vi "ClassSelectMess.vi"(7 "NewFunction":string, 8 "ErrorIn(No Error)":errorcluster caption="entrée d'erreur (pas d'erreur)", 9 "Text":string[][](array[string]), 10 "Functions":string[][](array[string]), 11 "Classes":string[][](array[string])) -> (0 "sortie d'erreur":errorcluster, 1 "CancelOut":bool, 2 "New":bool, 3 "InstrNameOut":string, 4 "Classindex":i32)   [LabVIEW 2019]
panel:
  out "Init Prog":bool
  in  "Cancel":bool
  in  "New":bool
  in  "Add":bool
  in  "LoadedDev":string(tree)
  # "Select an Instrument to add the function to or choose \"New\" to create the function into a new instrument"
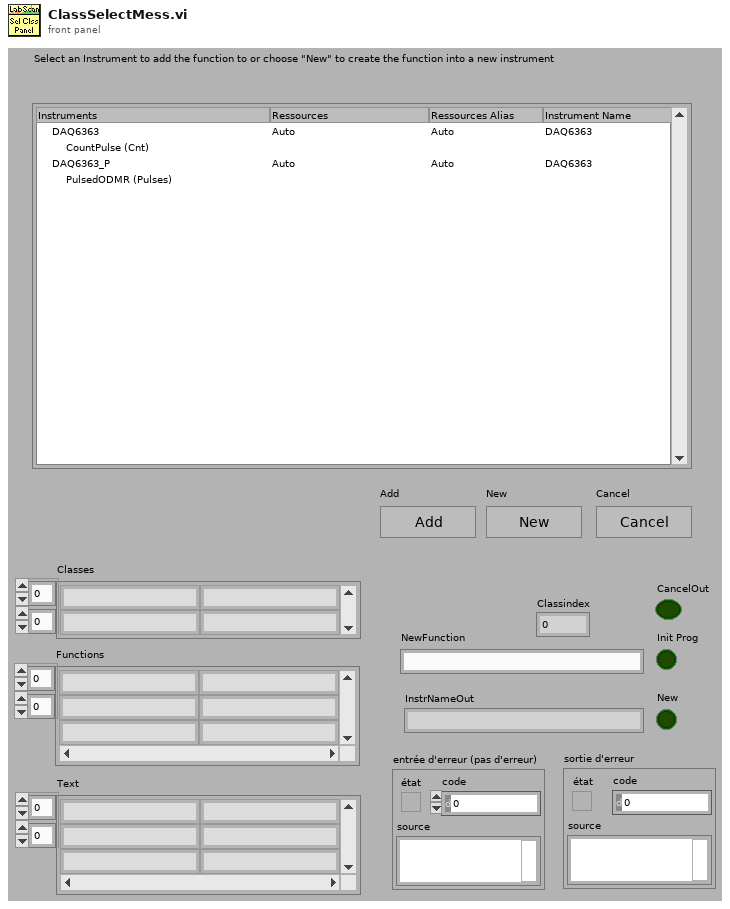
[diagram p1: front panel]
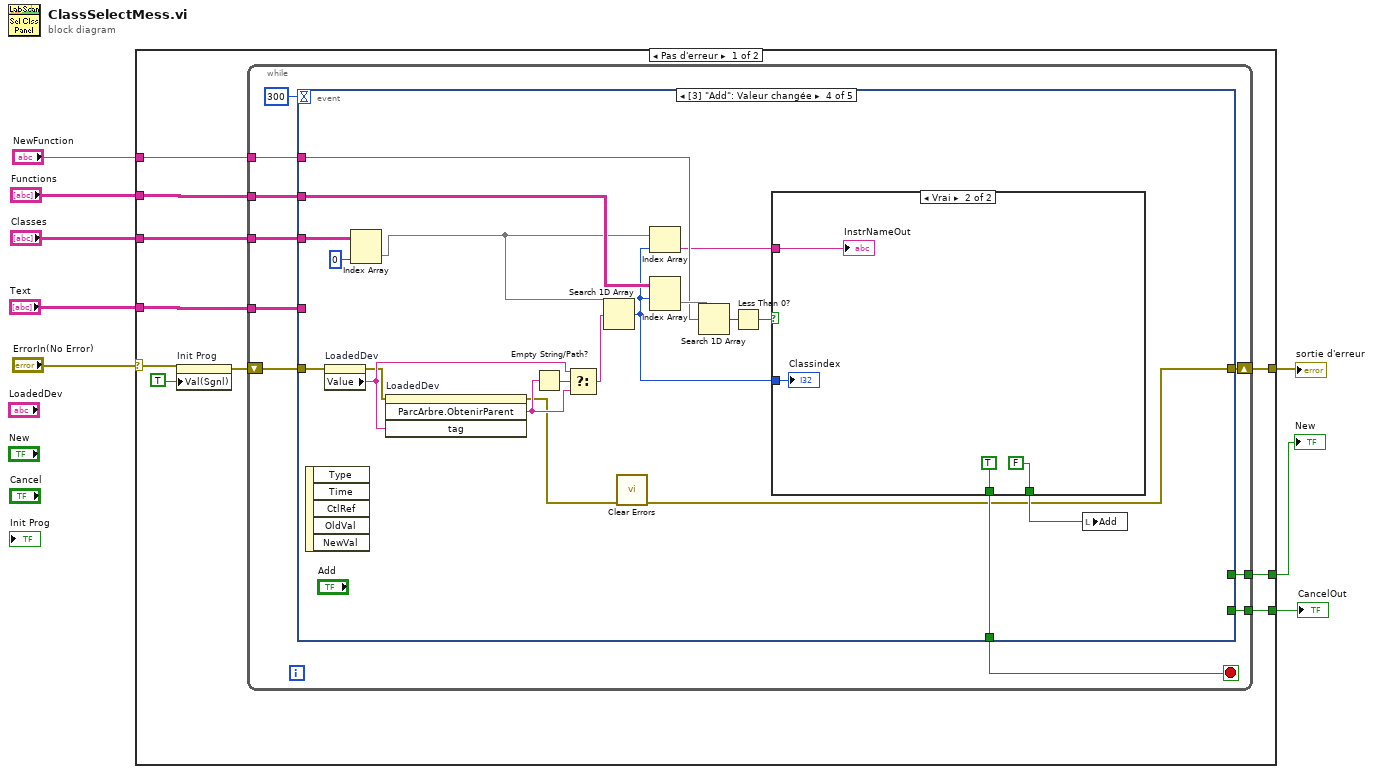
[diagram p0: block diagram]
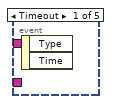
[diagram p2: hidden frame]
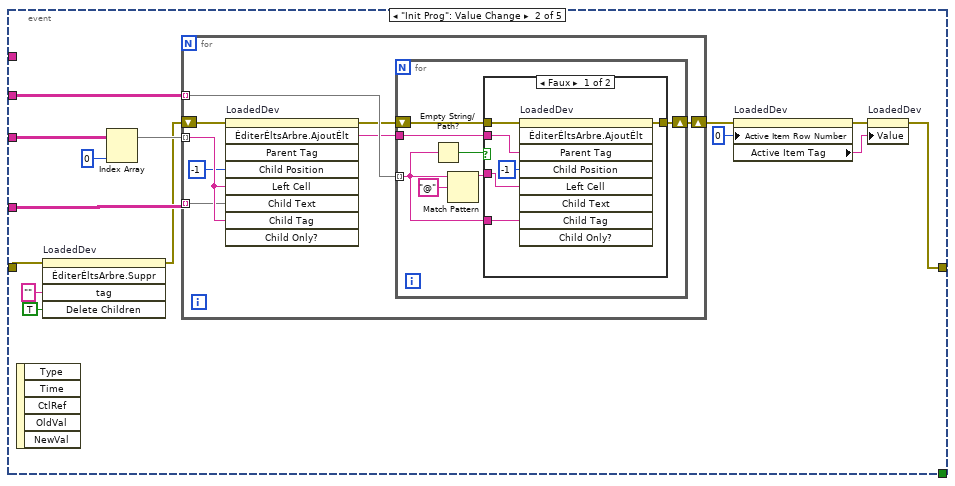
[diagram p3: hidden frame]
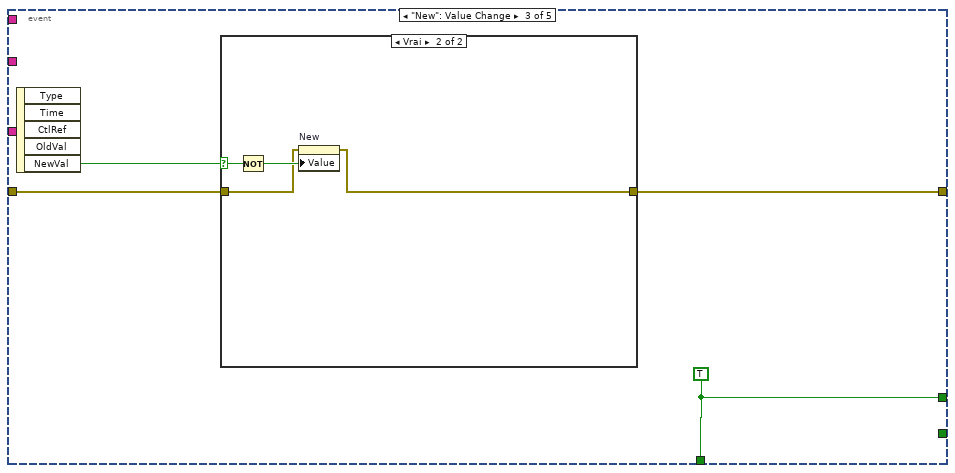
[diagram p5: hidden frame]
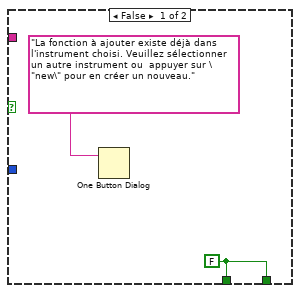
[diagram p7: hidden frame]
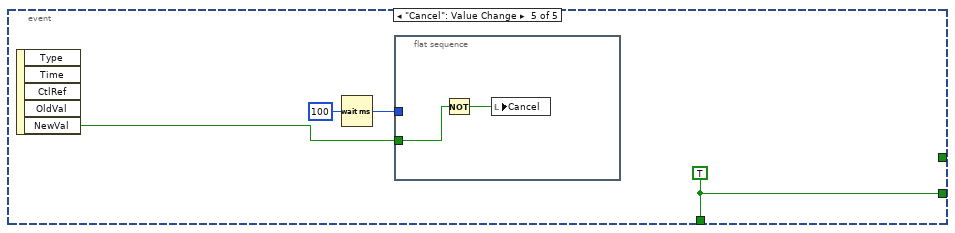
[diagram p8: hidden frame]
diagram:
  n1 = case shown="Pas d'erreur" "ErrorIn(No Error)" {
    selector: "ErrorIn(No Error)" -> [w14 w106]
    tunnel: "Classes" -> [w18 _]
    tunnel: "Functions" -> [w17 _]
    tunnel: "Text" -> [w16 _]
    tunnel: [w12 w106] -> w4
    tunnel: "NewFunction" -> [w11 _]
    tunnel: [w10 _] -> w2
    tunnel: [w9 _] -> w1
    frame No Error {
      n2 = property on="Init Prog" class="Bool (strict)"(error in=w14, "Val(Sgnl)"=TRUE ("Valeur (Signalisation)")) -> (error out=w13:errorcluster)  [unwired: 1 in, 1 out]
      n3 = while {
        tunnel: w18 -> [w28]
        tunnel: w17 -> [w27]
        tunnel: w16 -> [w26]
        shift-right: [w21] -> w12
        shift-left: w13 -> [w24]
        tunnel: w11 -> [w23]
        tunnel: [w20] -> w10
        tunnel: [w19] -> w9
        stop <- w22 stop-if-true
        n4 = event shown="[3] \"Add\": Valeur changée" {
          selector: _ -> [_ _ _ _ _]
          dyn-events: _ -> [_ _ _ _ _]
          timeout: 300 -> [_ _ _ _ _]
          tunnel: w28 -> [_ w41 _ w92 _]
          tunnel: w27 -> [_ w40 _ w91 _]
          tunnel: w26 -> [_ w42 _ _ _]
          tunnel: w24 -> [_ w37 w66 w93 _]
          tunnel: w23 -> [_ _ _ w89 _]
          tunnel: [_ _ w68 w86 w100] -> w22
          tunnel: [_ w33 w65 w75 _] -> w21
          tunnel: [_ _ w68 _ _] -> w20
          tunnel: [_ _ _ _ w100] -> w19
          event Timeout {
            n5 = event-data() -> ()  [unwired: 1 in, 2 out]
          }
          event "Init Prog": Value Change {
            n6 = event-data() -> ()  [unwired: 1 in, 5 out]
            n7 = invoke on="LoadedDev" class="Arbre (strict)" method="ÉditerÉltsArbre.Suppr"(error in=w37, "tag"="" ("Tag"), "Delete Children"=TRUE ("Supprimer les enfants ?")) -> (error out=w34:errorcluster)  [unwired: 2 in, 4 out]
            n8 = Index Array(array=w41, index (col)=0 ("indice désactivé (col)")) -> (element=w39:string[])  [unwired: 1 in]
            n9 = for {
              tunnel: w39 -> [w50] mode=indexing
              tunnel: w40 -> [w48] mode=indexing
              tunnel: w42 -> [w49] mode=indexing
              shift-right: [w46] -> w31
              shift-left: w34 -> [w45]
              n10 = invoke on="LoadedDev" class="Arbre (strict)" method="ÉditerÉltsArbre.AjoutÉlt"(error in=w45, "Child Position"=-1 ("Position de l'enfant"), "Left Cell"=w50, "Child Text"=w49, "Child Tag"=w50) -> (error out=w44:errorcluster, "Edit Tree Items:Add Item"=w47:string)  [unwired: 4 in, 7 out]
              n11 = for {
                tunnel: w48 -> [w52] mode=indexing
                tunnel: w47 -> [w57]
                shift-right: [w56] -> w46
                shift-left: w44 -> [w55]
                n12 = Empty String/Path?(string/path=w52) -> (empty?=w54:bool)
                n13 = Match Pattern(string=w52, regular expression="@" ("expression régulière")) -> (before substring=w53:string)  [unwired: 1 in, 3 out]
                n14 = case shown="Faux" w54 {
                  tunnel: w53 -> [w63 _]
                  tunnel: w57 -> [w62 _]
                  tunnel: [w61 w64] -> w56
                  tunnel: w55 -> [w60 w64]
                  tunnel: w52 -> [w59 _]
                  frame False {
                    n15 = invoke on="LoadedDev" class="Arbre (strict)" method="ÉditerÉltsArbre.AjoutÉlt"(error in=w60, "Parent Tag"=w62, "Child Position"=-1 ("Position de l'enfant"), "Left Cell"=w63, "Child Tag"=w59) -> (error out=w61:errorcluster)  [unwired: 4 in, 8 out]
                  }
                  frame True {
                  }
                }
              }
            }
            n16 = property on="LoadedDev" class="Arbre (strict)"(error in=w31, "Active Item Row Number"=0 ("Élément actif : numéro de ligne")) -> (error out=w30:errorcluster, "Active Item Tag"=w29:string)  [unwired: 1 in, 1 out]
            n17 = property on="LoadedDev" class="Arbre (strict)"(error in=w30, "Value"=w29) -> (error out=w33:errorcluster)  [unwired: 1 in, 1 out]
          }
          event "New": Value Change {
            w68 = TRUE ("Add")
            n18 = event-data() -> ("NewVal"=w67:bool)  [unwired: 1 in, 4 out]
            n19 = case shown="Vrai" w67 {
              selector: w67 -> [_ w73]
              tunnel: w66 -> [w69 w71]
              tunnel: [w69 w70] -> w65
              frame False {
              }
              frame True {
                n20 = Not(x=w73) -> (.not. x?=w72:bool)
                n21 = property on="New" class="Bool (strict)"(error in=w71, "Value"=w72) -> (error out=w70:errorcluster)  [unwired: 1 in, 1 out]
              }
            }
          }
          event "Add": Value Change {
            n22 = event-data() -> ()  [unwired: 1 in, 5 out]
            n23 = property on="LoadedDev" class="Arbre (strict)"(error in=w93) -> (error out=w77:errorcluster, "Value"=w81:string)  [unwired: 1 in, 1 out]
            n24 = Index Array(array=w92, index (col)=0 ("indice désactivé (col)")) -> (element=w79:string[])  [unwired: 1 in]
            n25 = invoke on="LoadedDev" class="Arbre (strict)" method="ParcArbre.ObtenirParent"(error in=w77, "tag"=w81) -> (error out=w76:errorcluster, "Navigate Tree:Get Parent"=w82:string)  [unwired: 2 in, 2 out]
            n26 = Empty String/Path?(string/path=w82) -> (empty?=w83:bool)
            n27 = Select(t=w81, s=w83, f=w82) -> (s? t:f=w80:string)
            n28 = Search 1D Array(1D array=w79, element=w80) -> (index of element=w74:i32)  [unwired: 1 in]
            n29 = call <vilib>:"Clear Errors.vi"("error in (no error)"=w76) -> ("error out"=w75:errorcluster)  [unwired: 5 in, 1 out]
            n30 = Index Array(array=w79, index=w74) -> (element=w84:string)
            n31 = Index Array(array=w91, index (row)=w74) -> (element=w90:string[])  [unwired: 1 in]
            n32 = Search 1D Array(1D array=w90, element=w89) -> (index of element=w87:i32)  [unwired: 1 in]
            n33 = Less Than 0?(x=w87) -> (x < 0?=w88:bool)
            n34 = case shown="Vrai" w88 {
              tunnel: [w94 TRUE ("Add")] -> w86
              tunnel: [w94 FALSE ("Add")] -> w78
              tunnel: w84 -> [_ w97]
              tunnel: w74 -> [_ w96]
              frame False {
                w94 = FALSE ("Add")
                n35 = One Button Dialog(message="La fonction à ajouter existe déjà dans l'instrument choisi. Veuillez sélectionner un autre instrument ou  appuyer sur \"new\" pour en créer un nouveau.") -> ()  [unwired: 1 in, 1 out]
              }
              frame True {
                "InstrNameOut" <- w97
                "Classindex" <- w96
              }
            }
            n36 = local write "Add"(w78) -> ()
          }
          event "Cancel": Value Change {
            w100 = TRUE ("Add")
            n37 = event-data() -> ("NewVal"=w101:bool)  [unwired: 1 in, 4 out]
            n38 = Wait (ms)(milliseconds to wait=u32 100 ("attente (ms)")) -> (millisecond timer value=w103:u32)
            n39 = flat-sequence {
              tunnel: w103 -> [_]
              tunnel: w101 -> [w105]
              frame #0 {
                n40 = Not(x=w105) -> (.not. x?=w104:bool)
                n41 = local write "Cancel"(w104) -> ()
              }
            }
          }
        }
      }
    }
    frame Error {
    }
  }
  "sortie d'erreur" <- w4
  "New" <- w2
  "CancelOut" <- w1
